vi "IR120917 selection supercontinuum_SD.vi"(1 "DATA":dbl[](array[numeric])) -> (0 "résultat selec SC":dbl[](array[numeric]))   [LabVIEW 2015]
uses:
  globalVarSD.vi
panel:
  out "Graphe":dbl[](graph)
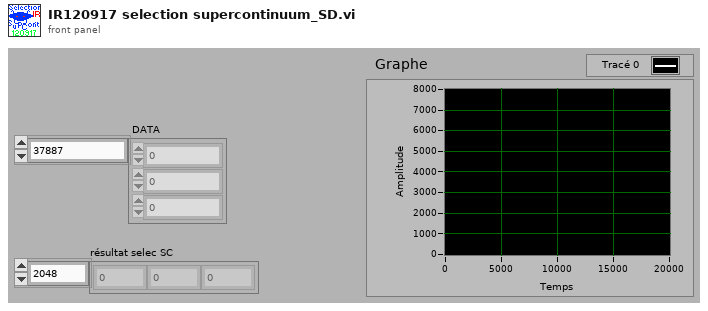
[diagram p1: front panel]
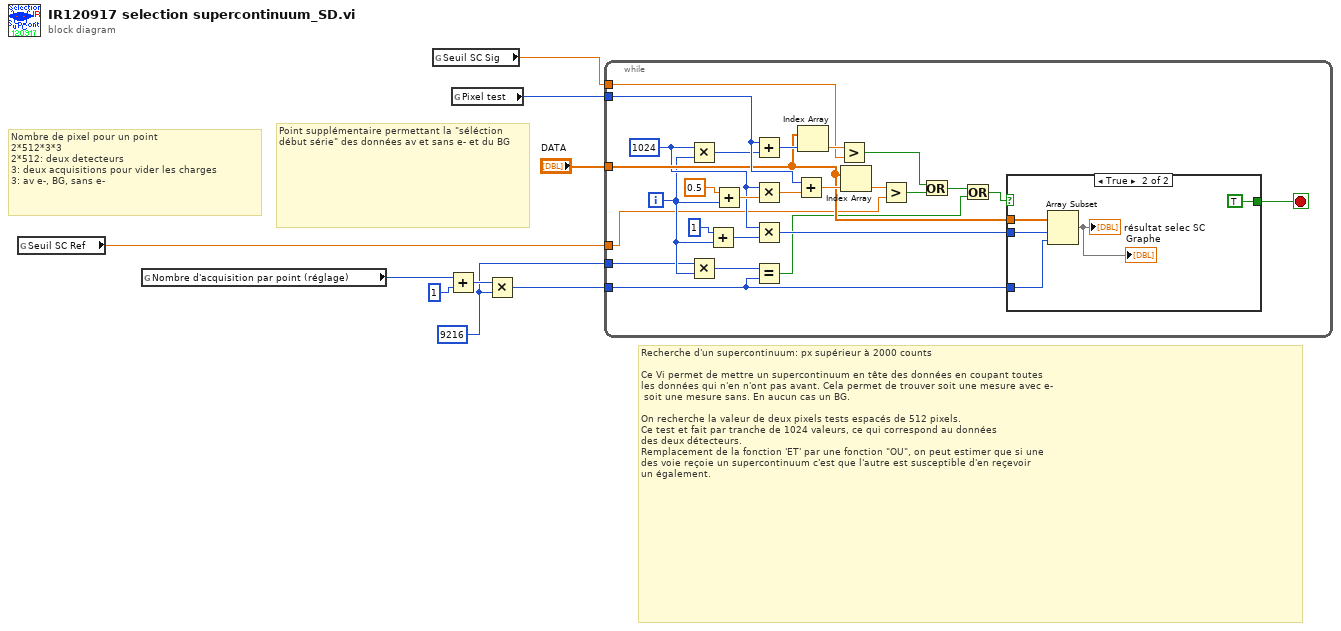
[diagram p0: block diagram]
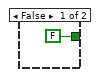
[diagram p2: hidden frame]
diagram:
  w5 = 9216 ("y")
  # "Nombre de pixel pour un point\n2*512*3*3\n2*512: deux detecteurs\n3: deux acquisitions pour vider les charges\n3: av e-, BG, sans e-"
  # "Recherche d'un supercontinuum: px supérieur à 2000 counts\n\nCe Vi permet de mettre un supercontinuum en tête des données en coupant toutes\nles données qui n'en n'ont pas avant. Cela permet de trouver soit une mesure avec e- \n soit une mesure sans. En aucun cas un BG.\n\nOn recherche la valeur de deux pixels tests espacés de 512 pixels.\nCe test et fait par tranche de 1024 valeurs, ce qui correspond au données\ndes deux détecteurs. \nRemplacement de la fonction 'ET' par une fonction \"OU\", on peut estimer que si une \ndes voie reçoie un supercontinuum c'est que l'autre est susceptible d'en reçevoir \nun également."
  # "Point supplémentaire permettant la \"séléction début série\" des données av et sans e- et du BG"
  n1 = global read "globalVarSD.vi" "Seuil SC Ref"() -> (w2:dbl)
  n2 = global read "globalVarSD.vi" "Nombre d'acquisition par point (réglage)"() -> (w3:u32)
  n3 = global read "globalVarSD.vi" "Seuil SC Sig"() -> (w1:dbl)
  n4 = Add(x=w3, y=1) -> (x+y=w9:u32)
  n5 = global read "globalVarSD.vi" "Pixel test"() -> (w4:u32)
  n6 = Multiply(x=w9, y=w5) -> (x*y=w6:u32)
  n7 = while {
    tunnel: w4 -> [w31]
    tunnel: "DATA" -> [w25]
    tunnel: w6 -> [w15]
    tunnel: w5 -> [w16]
    tunnel: w1 -> [w11]
    tunnel: w2 -> [w10]
    i -> [w17]
    stop <- w23 stop-if-true
    w20 = 1024 ("x")
    n8 = Multiply(x=w20, y=w17) -> (x*y=w24:i32)
    n9 = Multiply(x=w16, y=w17) -> (x*y=w14:i32)
    n10 = Add(x=1, y=w17) -> (x+y=w21:i32)
    n11 = Add(x=0.5, y=w17) -> (x+y=w29:dbl)
    n12 = Add(x=w31, y=w24) -> (x+y=w27:u32)
    n13 = Multiply(x=w20, y=w29) -> (x*y=w28:dbl)
    n14 = Multiply(x=w20, y=w21) -> (x*y=w19:i32)
    n15 = Equal?(x=w14, y=w15) -> (x = y?=w12:bool)
    n16 = Add(x=w31, y=w28) -> (x+y=w26:dbl)
    n17 = Index Array(array=w25, index=w27) -> (element=w35:dbl)
    n18 = Greater?(x=w35, y=w11) -> (0:w33:bool)
    n19 = Index Array(array=w25, index=w26) -> (element=w34:dbl)
    n20 = Greater?(x=w34, y=w10) -> (0:w32:bool)
    n21 = Or(x=w33, y=w32) -> (x .or. y?=w13:bool)
    n22 = Or(x=w13, y=w12) -> (x .or. y?=w18:bool)
    n23 = case shown="True" w18 {
      tunnel: w25 -> [_ w41]
      tunnel: w15 -> [_ w40]
      tunnel: w19 -> [_ w39]
      tunnel: [FALSE TRUE] -> w23
      frame False {
      }
      frame True {
        n24 = Array Subset(array=w41, index=w39, length=w40) -> (→"résultat selec SC" →"Graphe":dbl[])
      }
    }
  }
